vi "GetReleases.vi"(11 "GitHub":bool) -> (2 "Info":T1, 3 "infoReleases":T2)   [LabVIEW 2017]
uses:
  a7ec9648-ff3c-4189-9ce3-e5ab43f7bae3.vi
  <vilib>/JDP Science/JSONtext/JSON text to Variant.vi
  <vilib>/JDP Science/JSONtext/LVClass Serializer/JSONtext LVClass Serializer.lvclass
  <vilib>/httpClient/LabVIEWHTTPClient.lvlib
panel:
  in  "Cluster - Thin Border":T2
  out "headers":string
  out "body":string
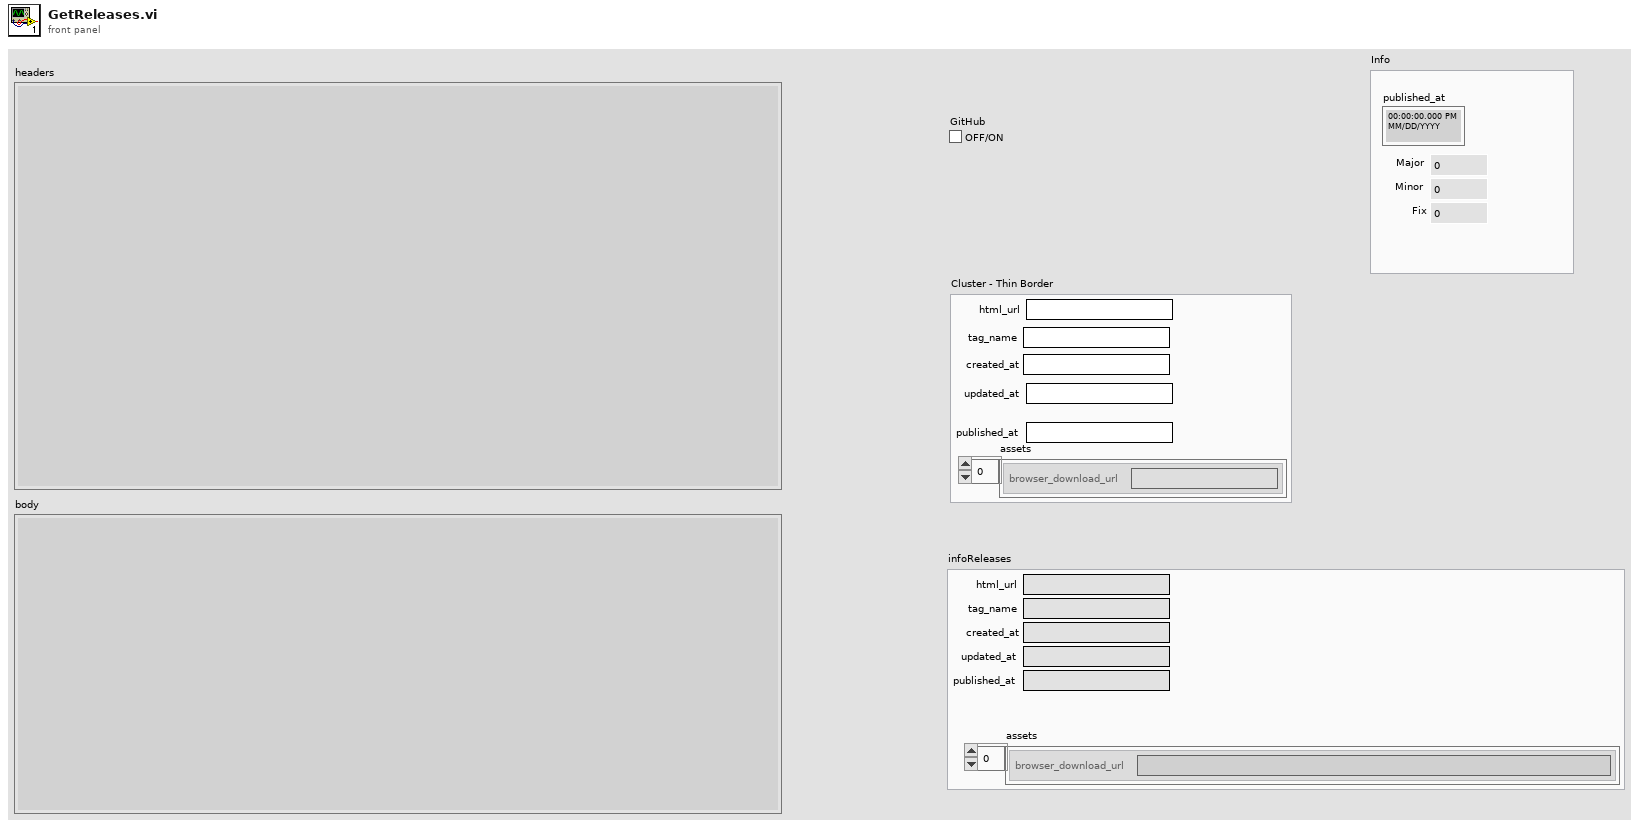
[diagram p1: front panel]
types:
  T1 = cluster{"published_at":timestamp, "Major":u32, "Minor":u32, "Fix":u32}
  T2 = cluster{"tag_name":string, "created_at":string, "updated_at":string, "published_at":string, "assets":cluster{"browser_download_url":string}[], "html_url":string}
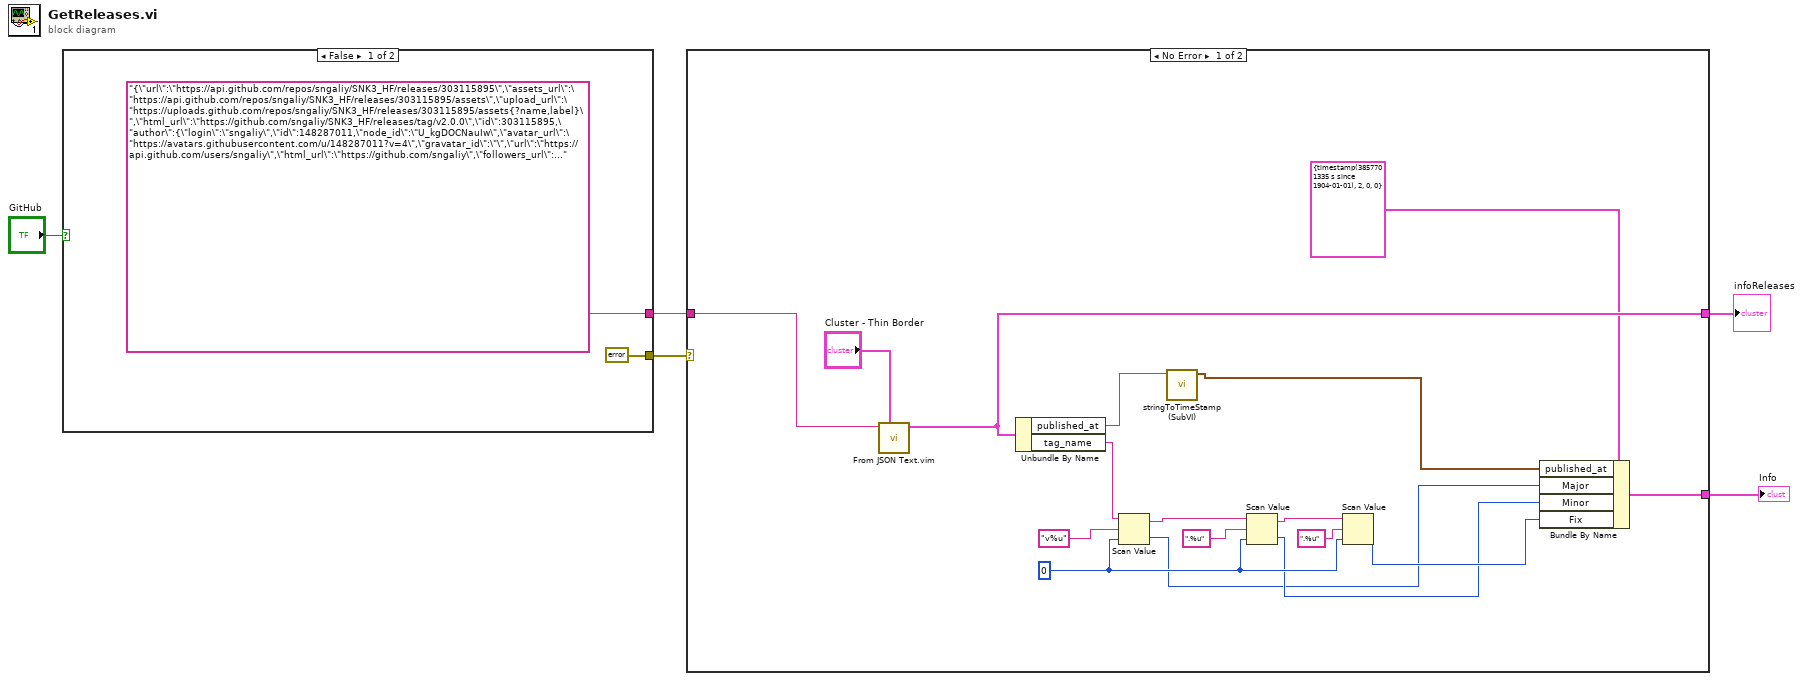
[diagram p0: block diagram]
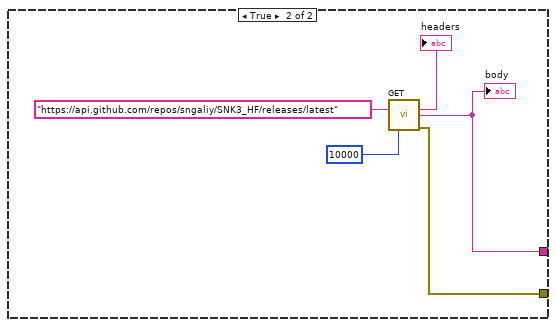
[diagram p2: hidden frame]
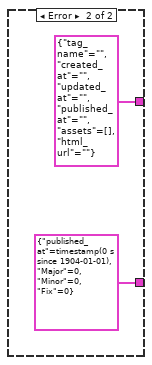
[diagram p3: hidden frame]
diagram:
  n1 = case shown="False" "GitHub" {
    tunnel: ["{\"url\":\"https://api.github.com/repos/sngaliy/SNK3_HF/releases/303115895\",\"assets_url\":\"https://api.github.com/repos/sngaliy/SNK3_HF/releases/303115895/assets\",\"upload_url\":\"https://uploads.github.com/repos/sngaliy/SNK3_HF/releases/303115895/assets{?name,label}\",\"html_url\":\"https://github.com/sngaliy/SNK3_HF/releases/tag/v2.0.0\",\"id\":303115895,\"author\":{\"login\":\"sngaliy\",\"id\":148287011,\"node_id\":\"U_kgDOCNauIw\",\"avatar_url\":\"https://avatars.githubusercontent.com/u/148287011?v=4\",\"gravatar_id\":\"\",\"url\":\"https://api.github.com/users/sngaliy\",\"html_url\":\"https://github.com/sngaliy\",\"followers_url\":\"https://api.github.com/users/sngaliy/followers\",\"following_url\":\"https://api.github.com/users/sngaliy/following{/other_user}\",\"gists_url\":\"https://api.github.com/users/sngaliy/gists{/gist_id}\",\"starred_url\":\"https://api.github.com/users/sngaliy/starred{/owner}{/repo}\",\"subscriptions_url\":\"https://api.github.com/users/sngaliy/subscriptions\",\"organizations_url\":\"https://api.github.com/users/sngaliy/orgs\",\"repos_url\":\"https://api.github.com/users/sngaliy/repos\",\"events_url\":\"https://api.github.com/users/sngaliy/events{/privacy}\",\"received_events_url\":\"https://api.github.com/users/sngaliy/received_events\",\"type\":\"User\",\"user_view_type\":\"public\",\"site_admin\":false},\"node_id\":\"RE_kwDOR0gGwM4SES53\",\"tag_name\":\"v1.8.8\",\"target_commitish\":\"main\",\"name\":\"Test1\",\"draft\":false,\"immutable\":true,\"prerelease\":false,\"created_at\":\"2026-03-30T10:28:47Z\",\"updated_at\":\"2026-03-30T10:42:16Z\",\"published_at\":\"2026-03-30T10:42:15Z\",\"assets\":[{\"url\":\"https://api.github.com/repos/sngaliy/SNK3_HF/releases/assets/384641176\",\"id\":384641176,\"node_id\":\"RA_kwDOR0gGwM4W7SiY\",\"name\":\"SNK3_HF_2.0.0.zip\",\"label\":null,\"uploader\":{\"login\":\"sngaliy\",\"id\":148287011,\"node_id\":\"U_kgDOCNauIw\",\"avatar_url\":\"https://avatars.githubusercontent.com/u/148287011?v=4\",\"gravatar_id\":\"\",\"url\":\"https://api.github.com/users/sngaliy\",\"html_url\":\"https://github.com/sngaliy\",\"followers_url\":\"https://api.github.com/users/sngaliy/followers\",\"following_url\":\"https://api.github.com/users/sngaliy/following{/other_user}\",\"gists_url\":\"https://api.github.com/users/sngaliy/gists{/gist_id}\",\"starred_url\":\"https://api.github.com/users/sngaliy/starred{/owner}{/repo}\",\"subscriptions_url\":\"https://api.github.com/users/sngaliy/subscriptions\",\"organizations_url\":\"https://api.github.com/users/sngaliy/orgs\",\"repos_url\":\"https://api.github.com/users/sngaliy/repos\",\"events_url\":\"https://api.github.com/users/sngaliy/events{/privacy}\",\"received_events_url\":\"https://api.github.com/users/sngaliy/received_events\",\"type\":\"User\",\"user_view_type\":\"public\",\"site_admin\":false},\"content_type\":\"application/x-zip-compressed\",\"state\":\"uploaded\",\"size\":8523694,\"digest\":\"sha256:af30a3c19c10c6b1866b233191b7098b6230e298d78d6251b4f5a4bb5a3b2531\",\"download_count\":2,\"created_at\":\"2026-03-30T10:39:51Z\",\"updated_at\":\"2026-03-30T10:39:55Z\",\"browser_download_url\":\"https://github.com/sngaliy/SNK3_HF/releases/download/v2.0.0/SNK3_HF_2.0.0.zip\"}],\"tarball_url\":\"https://api.github.com/repos/sngaliy/SNK3_HF/tarball/v2.0.0\",\"zipball_url\":\"https://api.github.com/repos/sngaliy/SNK3_HF/zipball/v2.0.0\",\"body\":\"\"}" ("body") w12] -> w4
    tunnel: [errorcluster {"status"=FALSE, "code"=0, "source"=""} ("error out") w8] -> w3
    frame False {
    }
    frame True {
      n2 = call <vilib>:"GET.vi"("url"="https://api.github.com/repos/sngaliy/SNK3_HF/releases/latest", "timeout (10000)"=10000) -> ("headers"=→"headers":string, "body"=w12:string, "error out"=w8:errorcluster)  [unwired: 10 in, 1 out]
      "body" <- w12
    }
  }
  n3 = case shown="No Error" w3 {
    tunnel: [w27 T2 {"tag_name"="", "created_at"="", "updated_at"="", "published_at"="", "assets"=[], "html_url"=""} ("Data out")] -> w5
    tunnel: w4 -> [w26 _]
    tunnel: [w16 T1 {"published_at"=timestamp(0 s since 1904-01-01), "Major"=0, "Minor"=0, "Fix"=0} ("Cluster - Thin Border 2")] -> w1
    frame No Error {
      w19 = u32 0 ("default (0 dbl)")
      n4 = call "From JSON Text.vim"("Data Type and Default Value"="Cluster - Thin Border", "JSON"=w26) -> ("Data out"=w27:T2)  [unwired: 8 in, 1 out]
      n5 = Unbundle By Name(w27) -> ("published_at"=w28:string, "tag_name"=w25:string)
      n6 = Scan Value(string=w25, format string="v%u", default (0 dbl)=w19) -> (output string=w23:string, value=w13:u32)
      n7 = call "stringToTimeStamp (SubVI).vi"("strTime"=w28) -> ("Time Stamp"=w17:timestamp)  [unwired: 10 in]
      n8 = Scan Value(string=w23, format string=".%u", default (0 dbl)=w19) -> (output string=w20:string, value=w14:u32)
      n9 = Scan Value(string=w20, format string=".%u", default (0 dbl)=w19) -> (value=w15:u32)  [unwired: 1 out]
      n10 = Bundle By Name(cluster=T1 {"published_at"=timestamp(3857701335 s since 1904-01-01), "Major"=2, "Minor"=0, "Fix"=0} ("Cluster - Thin Border 2"), "published_at"=w17, "Major"=w13, "Minor"=w14, "Fix"=w15) -> (w16:T1)
    }
    frame Error {
    }
  }
  "infoReleases" <- w5
  "Info" <- w1
